vi "tcp close.vi"(6 "length":i32, 7 "Array 2":string[](array[string]), 8 "error in":errorcluster, 9 "Address":i32, 10 "Write Data":sgl[](array[numeric])=[1.0, 1.0, 1.0, 1.0, 1.0, 1.0, 1.0, 1.0, 1.0, 1.0, 1.0, 1.0, 1.0, 1.0, 1.0, 100.0, 100.0, 100.0, 100.0, 100.0, 0.0, 100.0, 100.0, 100.0], 11 "connection ID IN":refnum<k5>) -> (0 "error out":errorcluster, 3 "connection ID out":refnum<k5>)   [LabVIEW 2015]
panel:
  out "String":string
  out "Array":string[](array[string])
  out "substring":string
  out "data out":string
  out "concatenated string":string
  out "Total Characters":i32
  out "Total Array":i32
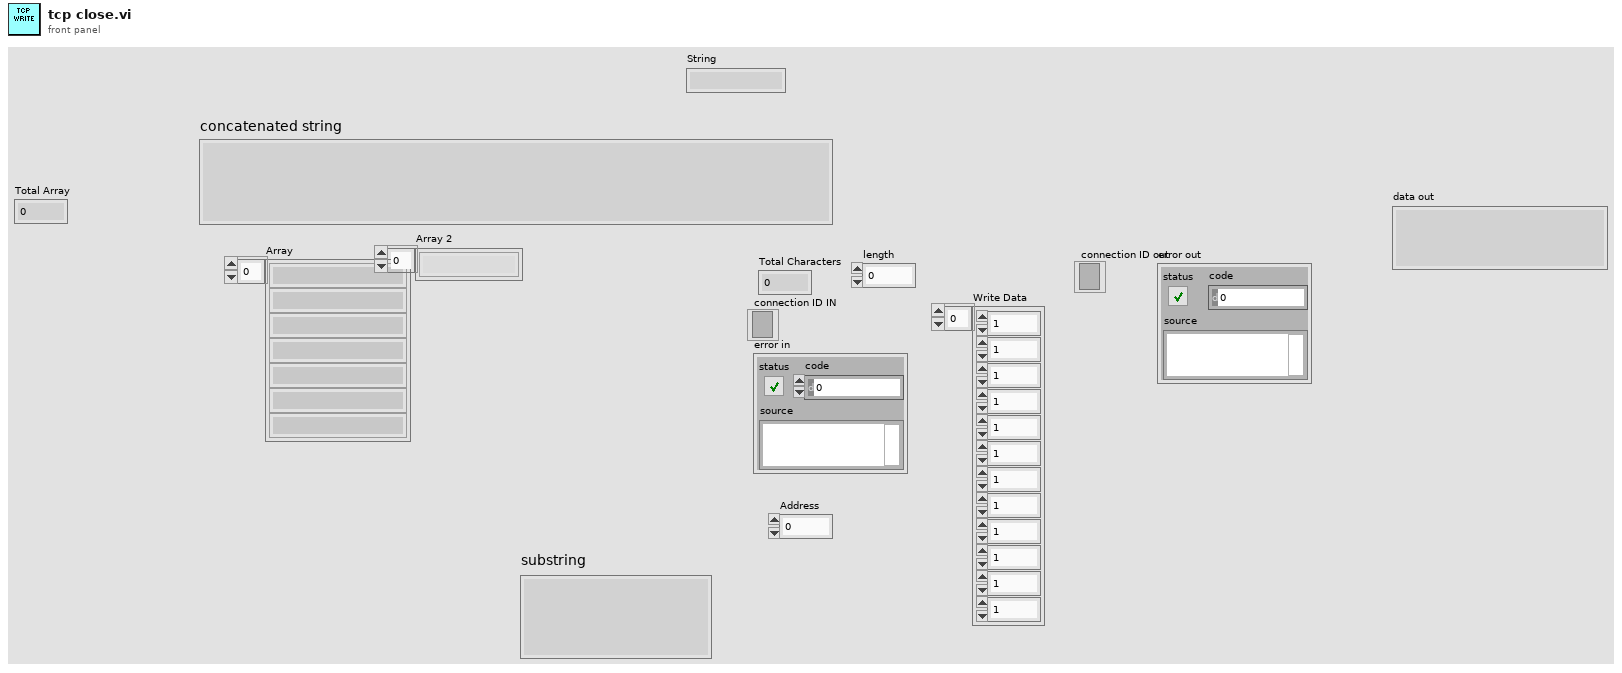
[diagram p1: front panel]
types:
  T1 = enum16{"Standard", "Buffered", "CRLF", "Immediate"}
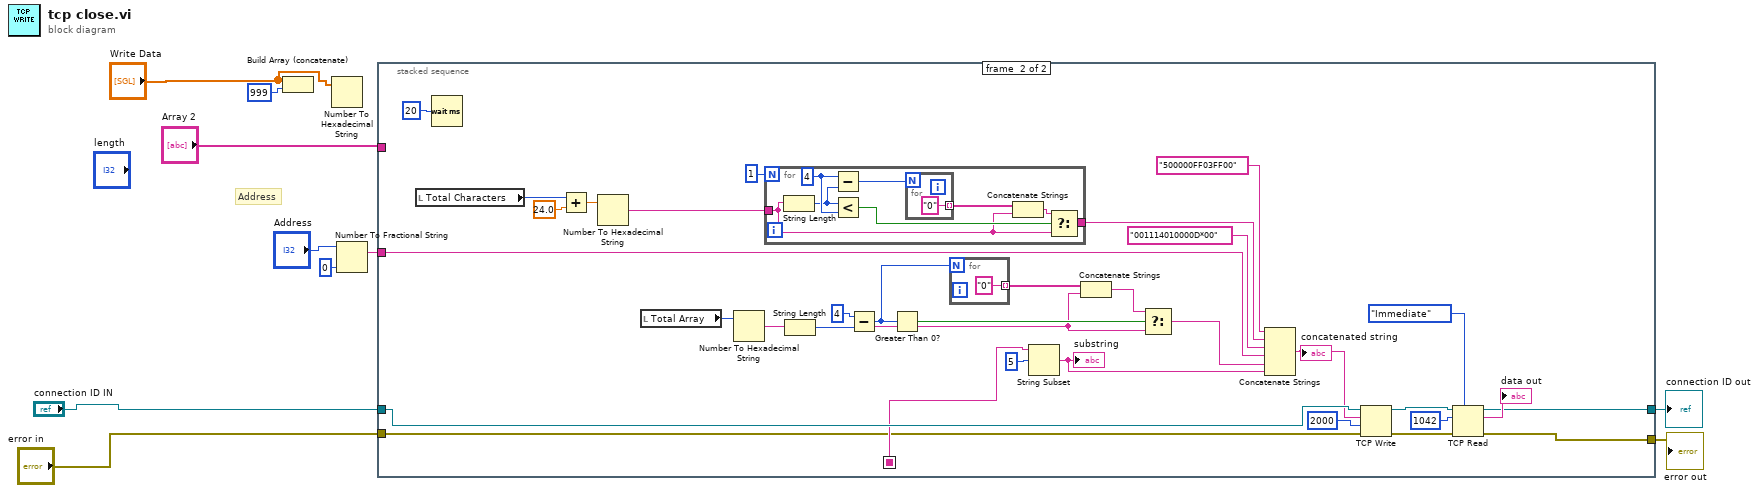
[diagram p0: block diagram]
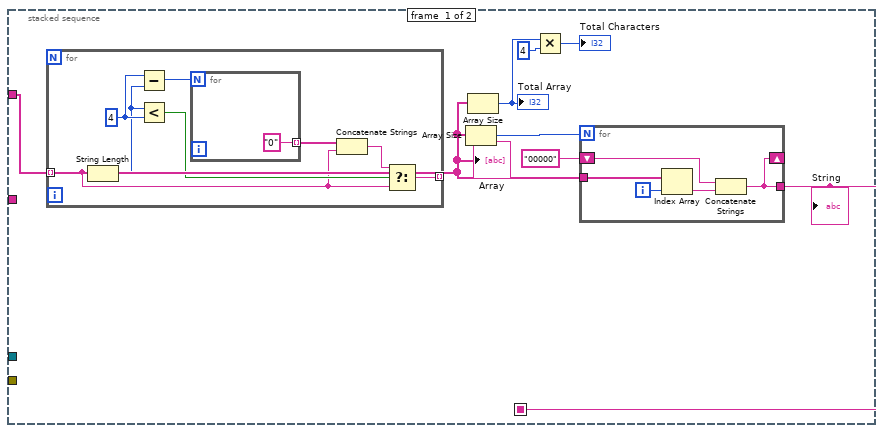
[diagram p2: hidden frame]
diagram:
  # "Address"
  n1 = Build Array (concatenate)("Write Data", 999) -> ()  [unwired: 1 out]
  n2 = Number To Hexadecimal String(2:"Write Data") -> ()  [unwired: 1 in, 1 out]
  n3 = Number To Fractional String(number="Address", precision (6)=i16 0) -> (F-format string=w5:string)  [unwired: 2 in]
  n4 = stacked-sequence {
    seq-local: [w16 _] -> [_ w62]
    tunnel: "connection ID IN" -> [_ w64]
    tunnel: "Array 2" -> [w11 _]
    tunnel: "error in" -> [_ w36]
    tunnel: [_ w35] -> w9
    tunnel: [_ w34] -> w8
    tunnel: w5 -> [_ w33]
    frame #0 {
      n5 = for {
        tunnel: w11 -> [w20] mode=indexing
        tunnel: [w18] -> _ mode=indexing
        w24 = 4 ("y")
        n6 = String Length(string=w20) -> (length=w23:i32)
        n7 = Subtract(x=w24, y=w23) -> (x-y=w22:i32)
        n8 = Less?(x=w23, y=w24) -> (x < y?=w25:bool)
        n9 = for {
          N: w22 -> [_]
          tunnel: ["0"] -> w21 mode=indexing
        }
        n10 = Concatenate Strings(w21, w20) -> (w19:string)
        n11 = Select(t=w19, s=w25, f=w20) -> (s? t:f=w18:string)
      }
      n12 = Array Size(array=w11) -> (size(s)=w15:i32)
      n13 = Array Size(array=w11) -> (size(s)=w12:i32)
      "Total Array" <- w12
      n14 = Multiply(x=w12, y=4) -> (x*y=→"Total Characters":i32)
      n15 = for {
        N: w15 -> [_]
        shift-right: [w29] -> _
        shift-left: "00000" -> [w28]
        tunnel: [w29] -> w16
        tunnel: w11 -> [w27]
        i -> [w31]
        n16 = Index Array(array=w27, index=w31) -> (element=w30:string)
        n17 = Concatenate Strings(w28, w30) -> (w29:string)
      }
      "String" <- w16
      "Array" <- w11
    }
    frame #1 {
      n18 = local read "Total Characters"() -> (w38:i32)
      n19 = Wait (ms)(milliseconds to wait=u32 20) -> ()  [unwired: 1 out]
      n20 = Add(x=w38, y=24.0) -> (x+y=w50:dbl)
      n21 = Number To Hexadecimal String(2:w50) -> (0:w51:string)  [unwired: 1 in]
      n22 = local read "Total Array"() -> (w37:i32)
      n23 = Number To Hexadecimal String(2:w37) -> (0:w56:string)  [unwired: 1 in]
      n24 = for {
        N: 1 -> [_]
        tunnel: w51 -> [w67]
        tunnel: [w65] -> w41
        w71 = 4 ("y")
        n25 = String Length(string=w67) -> (length=w70:i32)
        n26 = Subtract(x=w71, y=w70) -> (x-y=w69:i32)
        n27 = Less?(x=w70, y=w71) -> (x < y?=w72:bool)
        n28 = for {
          N: w69 -> [_]
          tunnel: ["0"] -> w68 mode=indexing
        }
        n29 = Concatenate Strings(w68, w67) -> (w66:string)
        n30 = Select(t=w66, s=w72, f=w67) -> (s? t:f=w65:string)
      }
      n31 = String Length(string=w56) -> (length=w60:i32)
      n32 = Subtract(x=4, y=w60) -> (x-y=w32:i32)
      n33 = Greater Than 0?(x=w32) -> (x > 0?=w58:bool)
      n34 = for {
        N: w32 -> [_]
        tunnel: ["0"] -> w46 mode=indexing
      }
      n35 = String Subset(string=w62, offset (0)=5) -> (substring=w47:string)  [unwired: 1 in]
      "substring" <- w47
      n36 = Concatenate Strings(w46, w56) -> (w57:string)
      n37 = Select(t=w57, s=w58, f=w56) -> (s? t:f=w40:string)
      n38 = Concatenate Strings("500000FF03FF00" ("data in"), w41, "001114010000D*00" ("data in"), w33, w40, w47) -> (w52:string)
      "concatenated string" <- w52
      n39 = TCP Write(connection ID=w64, data in=w52, error in (no error)=w36, 9:2000 ("timeout ms (25000)")) -> (connection ID out=w55:refnum<k5>, error out=w54:errorcluster)  [unwired: 1 out]
      n40 = TCP Read(connection ID=w55, bytes to read=1042, error in (no error)=w54, 7:T1."Immediate" ("mode (standard)")) -> (connection ID out=w35:refnum<k5>, data out=→"data out":string, error out=w34:errorcluster)  [unwired: 1 in]
    }
  }
  "connection ID out" <- w9
  "error out" <- w8
